vi "Find Missing.vi"(8 "new list in":T1[](array[typedef]) {"Creation Date" format="%<%x>T"; "Last Updated" format="%<%x>T"}, 11 "SR List in":T1[](array[typedef]) {"Creation Date" format="%<%x>T"; "Last Updated" format="%<%x>T"}) -> (3 "missing list out":T1[](array[typedef]) {"Creation Date" format="%<%x>T"; "Last Updated" format="%<%x>T"})   [LabVIEW 2018]
uses:
  Type Defs/SR Cluster.ctl
  Type Defs/SR Status.ctl
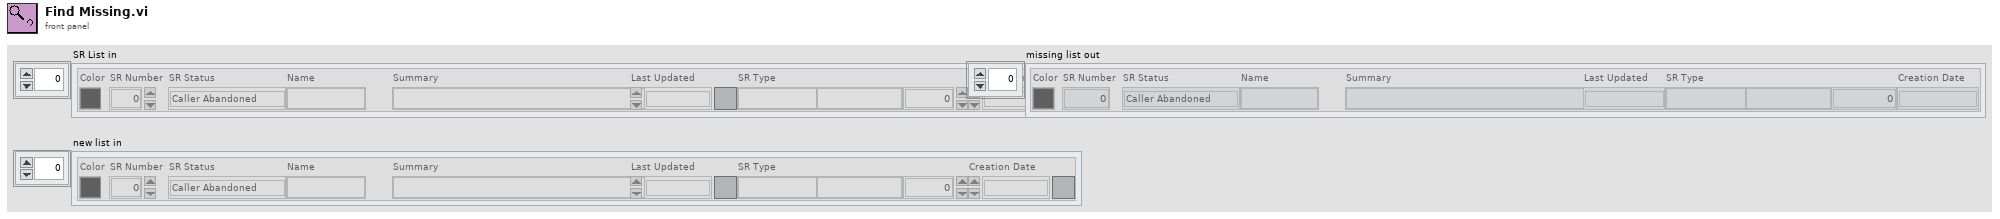
[diagram p1: front panel]
types:
  T1 = typedef "SR Cluster.ctl" = cluster{"Color":u32, "SR Number":i32, "SR Status":T2, "Name":string, "Summary":string, "Last Updated":timestamp, "SR Type":string, "Service Level":string, "Days Open":dbl, "Creation Date":timestamp}
  T2 = typedef "SR Status.ctl" = enum16{"Caller Abandoned", "Created in Error", "Expired", "Forum Resolved AE", "Forum Resolved Customer", "IN WORK", "IN WORK Collab with AES", "IN WORK Collab with PSE", "IN WORK Collab with SE", "IN WORK Customer Added Note", "IN WORK Escalation", "IN WORK Wait on Customer", "Open", "Potentially Resolved", "Presumed Resolved", "RMA Approved for Return", "Resolved", "Passed Off"}
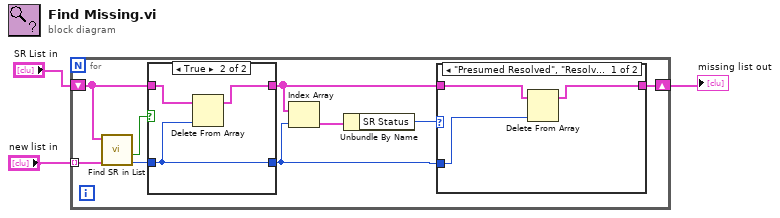
[diagram p0: block diagram]
diagram:
  n1 = for {
    tunnel: "new list in" -> [w10] mode=indexing
    shift-right: [w4] -> w1
    shift-left: "SR List in" -> [w9]
    n2 = call "Find SR in List.vi"("new SR"=w10, "SR list in"=w9) -> ("SR Index"=w11:i32, "Is SR in List?"=w12:bool)  [unwired: 8 in]
    n3 = case shown="True" w12 {
      tunnel: w11 -> [w18 w19]
      tunnel: w9 -> [w17 w21]
      tunnel: [w17 w20] -> w5
      tunnel: [w18 w19] -> w6
      frame False {
      }
      frame True {
        n4 = Delete From Array(array=w21, index=w19) -> (array with subset deleted=w20:T1[])  [unwired: 1 in, 1 out]
      }
    }
    n5 = Index Array(array=w5, index=w6) -> (element=w8:T1)
    n6 = Unbundle By Name(w8) -> ("SR Status"=w7:T2)
    n7 = case shown="\"Presumed Resolved\", \"Resolved\", \"Passed Off\"" w7 {
      tunnel: w6 -> [w13 _]
      tunnel: w5 -> [w15 w16]
      tunnel: [w14 w16] -> w4
      frame "Presumed Resolved", "Resolved", "Passed Off" {
        n8 = Delete From Array(array=w15, index=w13) -> (array with subset deleted=w14:T1[])  [unwired: 1 in, 1 out]
      }
      frame Default {
      }
    }
  }
  "missing list out" <- w1
